vi "Update Tree.vi"(7 "Filter Fails?":bool, 8 "error in (no error)":errorcluster, 9 "Test Tree":refnum<vi>, 10 "Result Model":refnum<class "Result Model.lvclass">) -> (0 "error out":errorcluster)   [LabVIEW 2020, in "Execution UI.lvclass"]
uses:
  Execution UI.lvclass
  Result Model/Result Model.lvclass
  Result Model/Tree Item Filter.ctl
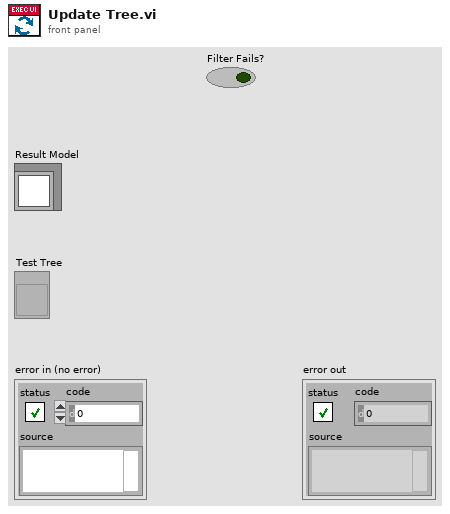
[diagram p1: front panel]
types:
  T1 = typedef "Result Model.lvclass/Tree Item Filter.ctl" = enum16{"All", "Only Fails", "Fails or else Not Executed"}
  T2 = cluster{"Left Cell String":string, "Child Text":string[], "Child Tag":string, "Item Indent":i32, "Child Only?":bool, "Glyph Index":i32}[]
  T3 = typedef "LVNodeAndColumnTypeDef.ctl" = cluster{"Node":string, "Column":i32}
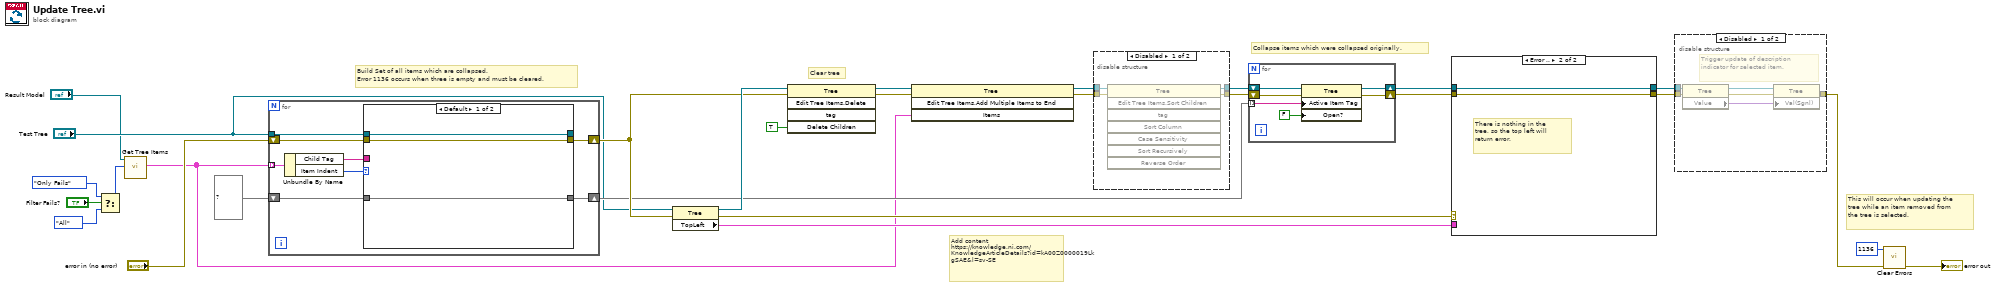
[diagram p0: block diagram]
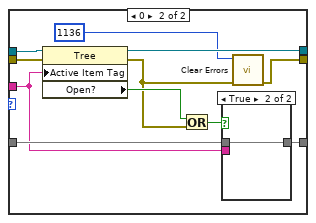
[diagram p4: hidden frame]
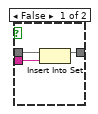
[diagram p5: hidden frame]
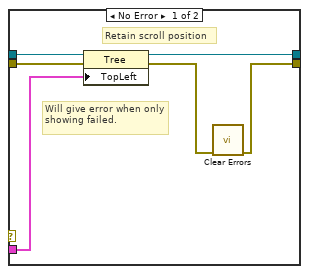
[diagram p6: hidden frame]
diagram:
  # "Collapse items which were collapsed originally."
  # "Build Set of all items which are collapsed.\nError 1136 occurs when three is empty and must be cleared."
  # "This will occur when updating the tree while an item removed from the tree is selected."
  # "Add content\nhttps://knowledge.ni.com/KnowledgeArticleDetails?id=kA00Z0000019LkgSAE&l=sv-SE"
  # "Clear tree"
  n1 = Select(t=Tree_Item_Filter."Only Fails" ("Filter"), s="Filter Fails?", f=Tree_Item_Filter."All" ("Filter")) -> (s? t:f=w2:T1)
  n2 = call "Get Tree Items.vi"("Filter"=w2, "Result Model by Reference In"="Result Model") -> ("Tree Items"=w7:T2)  [unwired: 8 in, 1 out]
  n3 = for {
    tunnel: w7 -> [w36] mode=indexing
    shift-right: [w30] -> w18
    shift-left: "error in (no error)" -> [w31]
    shift-right: [w33] -> w16
    shift-left: set{string} {} ("set") -> [w34]
    tunnel: "Test Tree" -> [w35]
    n4 = Unbundle By Name(w36) -> ("Child Tag"=w32:string, "Item Indent"=w29:i32)
    n5 = case shown="Default" w29 {
      tunnel: w35 -> [w38 w50]
      tunnel: [w38 w49] -> _
      tunnel: w34 -> [w39 w48]
      tunnel: [w39 w47] -> w33
      tunnel: w32 -> [_ w46]
      tunnel: w31 -> [w37 w44]
      tunnel: [w37 w43] -> w30
      frame Default {
      }
      frame 0 {
        n6 = property class="Tree"(reference=w50, error in=w44, "Active Item Tag"=w46) -> (reference out=w49:refnum<vi>, error out=w40:errorcluster, "Open?"=w45:bool)
        n7 = Or(x=w45, y=w40) -> (x .or. y?=w41:bool)
        n8 = case shown="True" w41 {
          tunnel: w48 -> [w53 w54]
          tunnel: [w52 w54] -> w47
          tunnel: w46 -> [w51 _]
          frame False {
            n9 = Insert Into Set(10:w51, 11:w53) -> (3:w52:set{string})  [unwired: 1 out]
          }
          frame True {
          }
        }
        n10 = call <vilib>:"Clear Errors.vi"("error in (no error)"=w40, "specific error code to clear (0: all)"=1136) -> ("error out"=w43:errorcluster)  [unwired: 4 in, 1 out]
      }
    }
  }
  n11 = property on="Property Node" class="Tree"(reference="Test Tree", error in=w18) -> (reference out=w25:refnum<vi>, error out=w24:errorcluster, "TopLeft"=w23:T3)
  n12 = invoke on="Invoke Node" class="Tree" method="Edit Tree Items.Delete"(reference=w25, error in=w18, "Delete Children"=TRUE ("Delete Children?")) -> (reference out=w27:refnum<vi>, error out=w26:errorcluster)  [unwired: 2 in, 3 out]
  n13 = invoke class="Tree" method="Edit Tree Items.Add Multiple Items to End"(reference=w27, error in=w26, "Items"=w7) -> (reference out=w13:refnum<vi>, error out=w9:errorcluster)  [unwired: 1 in, 2 out]
  n14 = disable-structure shown="Disabled" {
    disable-tunnel: w13 -> [w58 w60]
    disable-tunnel: [w57 w60] -> w10
    disable-tunnel: w9 -> [w56 w59]
    disable-tunnel: [w55 w59] -> w8
    frame Disabled {
      n15 = invoke class="Tree" method="Edit Tree Items.Sort Children"(reference=w58, error in=w56) -> (reference out=w57:refnum<vi>, error out=w55:errorcluster)  [unwired: 6 in, 6 out]
    }
    frame Enabled {
    }
  }
  n16 = for {
    shift-right: [w65] -> w12
    shift-left: w10 -> [w66]
    shift-right: [w64] -> w11
    shift-left: w8 -> [w63]
    tunnel: w16 -> [w62] mode=indexing
    n17 = property class="Tree"(reference=w66, error in=w63, "Active Item Tag"=w62, "Open?"=FALSE ("Active Item:Open?")) -> (reference out=w65:refnum<vi>, error out=w64:errorcluster)
  }
  n18 = case shown="Error .." w24 {
    tunnel: w12 -> [w72 w74]
    tunnel: [w71 w74] -> w15
    tunnel: w11 -> [w70 w73]
    tunnel: [w67 w73] -> w14
    tunnel: w23 -> [w68 _]
    frame No Error {
      # "Will give error when only showing failed."
      # "Retain scroll position"
      n19 = property on="Property Node" class="Tree"(reference=w72, error in=w70, "TopLeft"=w68) -> (reference out=w71:refnum<vi>, error out=w69:errorcluster)
      n20 = call <vilib>:"Clear Errors.vi"("error in (no error)"=w69) -> ("error out"=w67:errorcluster)  [unwired: 5 in, 1 out]
    }
    frame Error {
      # "There is nothing in the tree, so the top left will return error."
    }
  }
  n21 = disable-structure shown="Disabled" {
    disable-tunnel: [w78 w81] -> w22
    disable-tunnel: w15 -> [w76 _]
    disable-tunnel: w14 -> [w75 w81]
    frame Disabled {
      # "Trigger update of description indicator for selected item."
      n22 = property on="Property Node" class="Tree"(reference=w76, error in=w75) -> (reference out=w80:refnum<vi>, error out=w79:errorcluster, "Value"=w77:variant)
      n23 = property on="Property Node" class="Tree"(reference=w80, error in=w79, "Val(Sgnl)"=w77) -> (error out=w78:errorcluster)  [unwired: 1 out]
    }
    frame Enabled {
    }
  }
  n24 = call <vilib>:"Clear Errors.vi"("error in (no error)"=w22, "specific error code to clear (0: all)"=1136) -> ("error out"=→"error out":errorcluster)  [unwired: 4 in, 1 out]
